vi "get.vi"(8 "error in (no error)":errorcluster, 11 "Stresing_dual_cam in":refnum<class "Stresing_dual_cam.lvclass">) -> (0 "error out":errorcluster, 1 "data_raw_sig":u16[][](array[numeric]), 2 "data_raw_ref":u16[][](array[numeric]), 3 "Stresing_dual_cam out":refnum<class "Stresing_dual_cam.lvclass">, 4 "chop_sig":bool[](array[boolean]), 6 "chop_ref":bool[](array[boolean]))   [LabVIEW 2019, in "Stresing_dual_cam.lvclass"]
uses:
  Stresing_dual_cam.lvclass
  Stresing_dual_cam.lvclass/Stresing_dual_cam.ctl
  <vilib>/Analysis/baseanly.llb/Mean (DBL).vi
  <instrlib>/StresingDualCam/board.vis/Globals.vi
  <vilib>/Analysis/NI_AALBase.lvlib
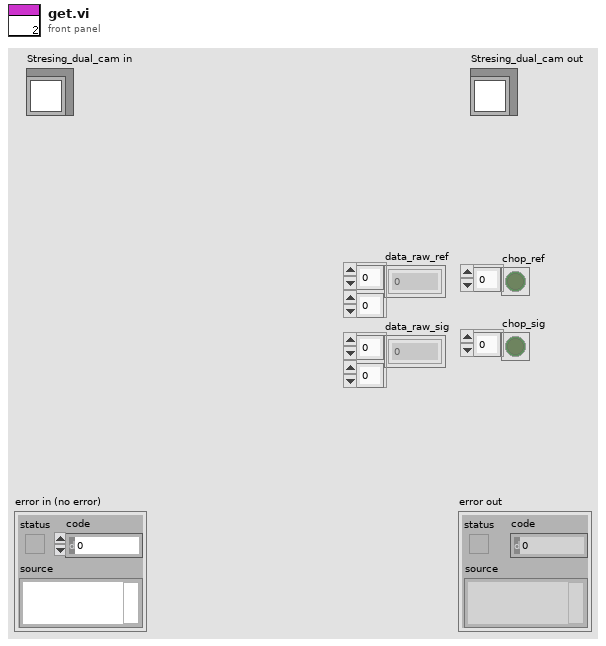
[diagram p1: front panel]
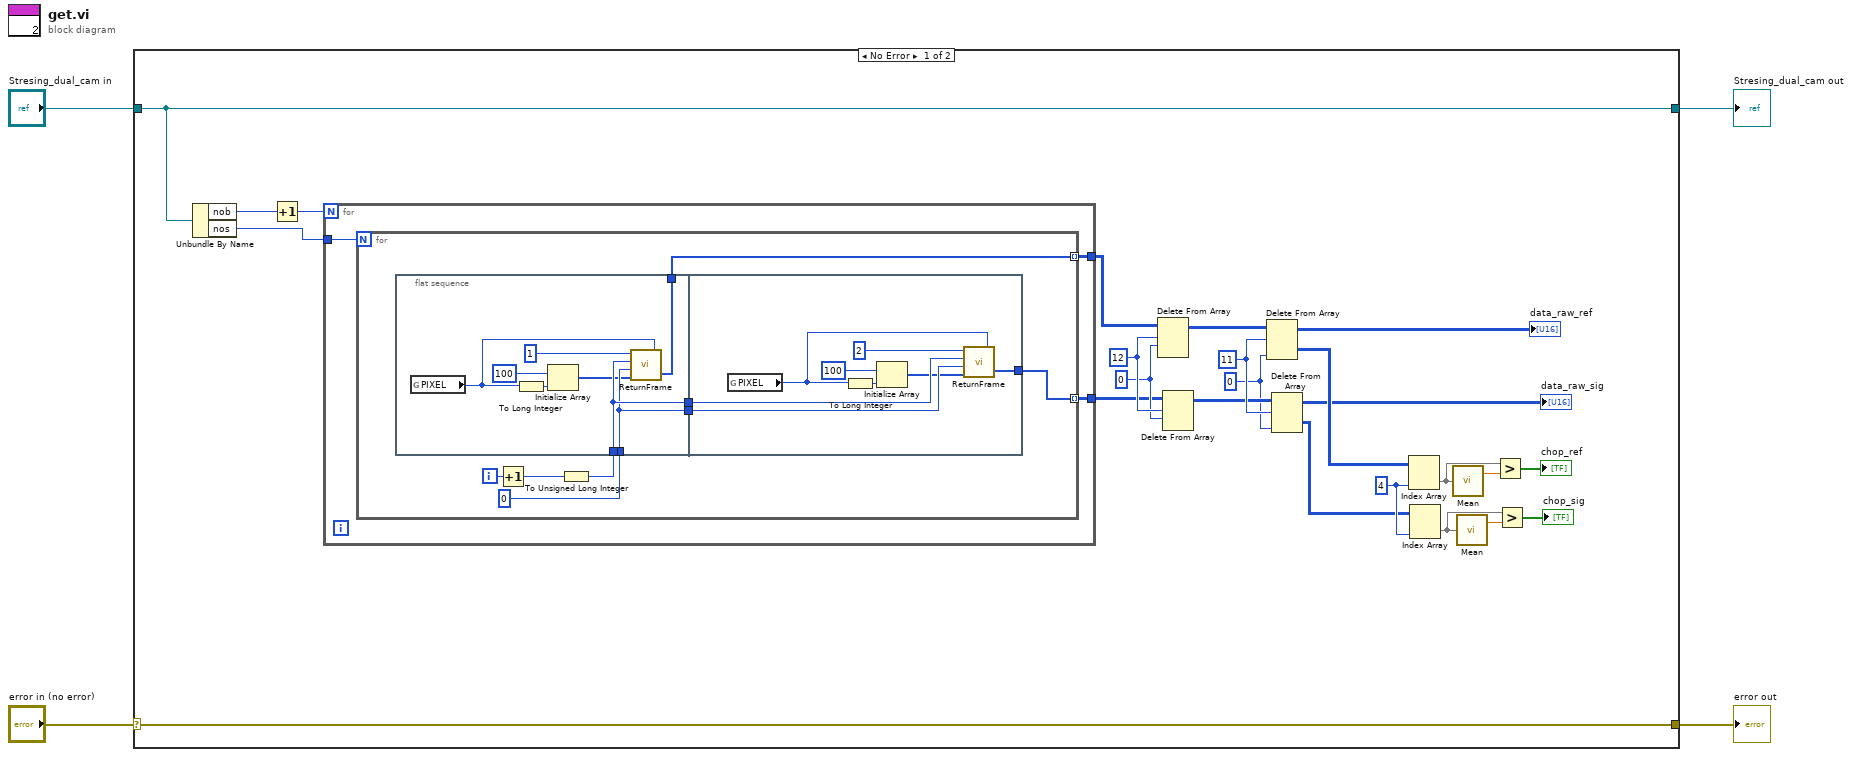
[diagram p0: block diagram]
diagram:
  n1 = case shown="No Error" "error in (no error)" {
    selector: "error in (no error)" -> [w28 w57]
    tunnel: [w28 w57] -> w3
    tunnel: [w27 w56] -> w1
    tunnel: "Stresing_dual_cam in" -> [w27 w56]
    frame No Error {
      w15 = 4
      w18 = 0
      w21 = 11 ("length")
      w22 = 0
      w23 = 12 ("length")
      n2 = Unbundle By Name(w27) -> ("nob"=w26:u32, "nos"=w24:u32)
      n3 = Increment(x=w26) -> (x+1=w25:u32)
      n4 = for {
        N: w25 -> [_]
        tunnel: [w31] -> w17
        tunnel: [w30] -> w16
        tunnel: w24 -> [w29]
        n5 = for {
          N: w29 -> [_]
          tunnel: [w39] -> w31 mode=indexing
          tunnel: [w35] -> w30 mode=indexing
          i -> [w37]
          n6 = flat-sequence {
            tunnel: [w41] -> w39
            tunnel: u32 0 -> [w43]
            tunnel: w36 -> [w44]
            tunnel: [w44] -> w34
            tunnel: [w43] -> w33
            tunnel: [w49] -> w35
            tunnel: w34 -> [w52]
            tunnel: w33 -> [w51]
            frame #0 {
              n7 = global read "Globals.vi" "PIXEL"() -> (w40:u32)
              n8 = To Long Integer(number=w40) -> (32bit integer=w46:i32)
              n9 = Initialize Array(u16 100, w46) -> (w42:u16[])
              n10 = call <instrlib>:"ReturnFrame.vi"("length"=w40, "Data Values In"=w42, "curr_nob"=w43, "curr_nos"=w44, "Drv"=u32 1) -> ("Data Values Out"=w41:u16[])
            }
            frame #1 {
              n11 = global read "Globals.vi" "PIXEL"() -> (w48:u32)
              n12 = To Long Integer(number=w48) -> (32bit integer=w55:i32)
              n13 = Initialize Array(u16 100, w55) -> (w50:u16[])
              n14 = call <instrlib>:"ReturnFrame.vi"("length"=w48, "Data Values In"=w50, "curr_nob"=w51, "curr_nos"=w52, "Drv"=u32 2) -> ("Data Values Out"=w49:u16[])
            }
          }
          n15 = Increment(x=w37) -> (x+1=w32:i32)
          n16 = To Unsigned Long Integer(number=w32) -> (unsigned 32bit integer=w36:u32)
        }
      }
      n17 = Delete From Array(array=w17, length=w23, index (row)=w22) -> (array with subset deleted=w20:u16[][])  [unwired: 1 in, 1 out]
      n18 = Delete From Array(array=w16, length=w23, index (row)=w22) -> (array with subset deleted=w19:u16[][])  [unwired: 1 in, 1 out]
      n19 = Delete From Array(array=w20, length=w21, index (col)=w18) -> (deleted portion=w10:u16[][], array with subset deleted=→"data_raw_ref":u16[][])  [unwired: 1 in]
      n20 = Delete From Array(array=w19, length=w21, index (col)=w18) -> (deleted portion=w9:u16[][], array with subset deleted=→"data_raw_sig":u16[][])  [unwired: 1 in]
      n21 = Index Array(array=w10, index (col)=w15) -> (element=w14:u16[])  [unwired: 1 in]
      n22 = Index Array(array=w9, index (col)=w15) -> (element=w11:u16[])  [unwired: 1 in]
      n23 = call-poly <vilib>:"Mean.vi"("X"=w14) -> ("mean"=w13:dbl)  [unwired: 1 out]
      n24 = call-poly <vilib>:"Mean.vi"("X"=w11) -> ("mean"=w12:dbl)  [unwired: 1 out]
      n25 = Greater?(x=w14, y=w13) -> (0:→"chop_ref":bool[])
      n26 = Greater?(x=w11, y=w12) -> (0:→"chop_sig":bool[])
    }
    frame Error {
    }
  }
  "error out" <- w3
  "Stresing_dual_cam out" <- w1
